vi "Connect Queue.vi"(8 "error in (no error)":errorcluster) -> (0 "error out":errorcluster, 3 "TCPConnection":refnum<class "LocalQueueConnection.lvclass">)   [LabVIEW 2013, in "MQTT_Queue.lvlib" / "LocalQueueConnection.lvclass"]
uses:
  LocalQueueConnection.lvclass
  MQTT_Connection/Connection/Connection.lvclass
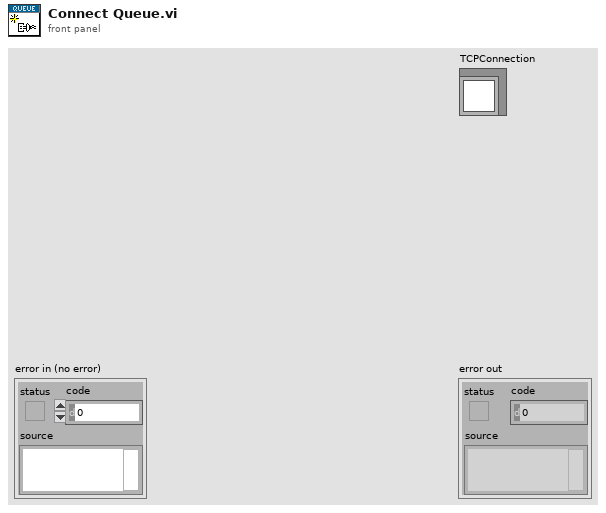
[diagram p1: front panel]
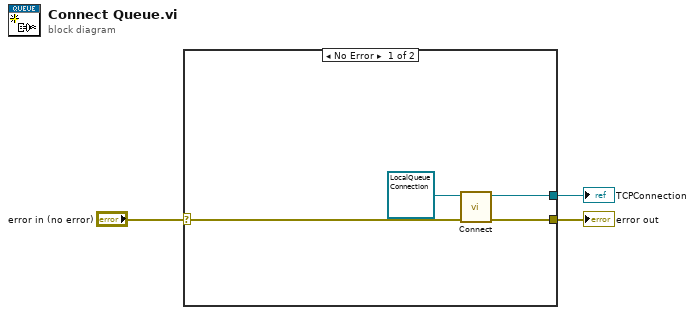
[diagram p0: block diagram]
diagram:
  n1 = case shown="No Error" "error in (no error)" {
    selector: "error in (no error)" -> [w4 w8]
    tunnel: [w6 w8] -> w2
    tunnel: [w7 _] -> w1
    frame No Error {
      n2 = call "Connect.vi"("error in (no error)"=w4, "Connection in"=refnum<class "LocalQueueConnection.lvclass"> refnum ("TCPConnection in")) -> ("error out"=w6:errorcluster, "Connection out"=w7:refnum<class "LocalQueueConnection.lvclass">)  [unwired: 8 in]
    }
    frame Error {
    }
  }
  "error out" <- w2
  "TCPConnection" <- w1
